vi "Start Acquisition and Logging.vi"(8 "error in (no error)":errorcluster, 11 "Acquisition and Logging Configuration":T1={"Data Rate"=1, "Samples per Read"=0, "Number of Reads to Save"=0, "Data File Name"="", "TDMS Properties"=[], "Number of Channels"=4, "Channel Scale Array"=[0.0, 0.0, 0.0, 0.0], "Channel Names"=[], "Trigger - RMS Value"=0.0, "Trigger - Channel"=0, "Trigger - Time (Minute)"=0} {"Data Rate" items=["51.200 kS/s (NI 9234)"=1, "25.600 kS/s (NI 9234)"=2, "17.067 kS/s (NI 9234)"=3, "12.800 kS/s (NI 9234)"=4, "10.240 kS/s (NI 9234)"=5, "8.533 kS/s (NI 9234)"=6, "7.314 kS/s (NI 9234)"=7, "6.400 kS/s (NI 9234)"=8, "5.689 kS/s (NI 9234)"=9, "5.120 kS/s (NI 9234)"=10, "4.654 kS/s (NI 9234)"=11, "4.267 kS/s (NI 9234)"=12, "3.938 kS/s (NI 9234)"=13, "3.657 kS/s (NI 9234)"=14, "3.413 kS/s (NI 9234)"=15, "3.200 kS/s (NI 9234)"=16, "3.012 kS/s (NI 9234)"=17, "2.845 kS/s (NI 9234)"=18, "2.695 kS/s (NI 9234)"=19, "2.560 kS/s (NI 9234)"=20, "2.438 kS/s (NI 9234)"=21, "2.328 kS/s (NI 9234)"=22, "2.226 kS/s (NI 9234)"=23, "2.133 kS/s (NI 9234)"=24, "2.048 kS/s (NI 9234)"=25, "1.969 kS/s (NI 9234)"=26, "1.896 kS/s (NI 9234)"=27, "1.829 kS/s (NI 9234)"=28, "1.765 kS/s (NI 9234)"=29, "1.707 kS/s (NI 9234)"=30, "1.652 kS/s (NI 9234)"=31]}) -> (0 "error out":errorcluster, 1 "Wait on IRQ Timeout?":bool, 2 "Total Buffer Size":i32, 3 "FPGA VI Reference Out":T4)   [LabVIEW 2020]
uses:
  controls/FPGA VI Reference.ctl
  controls/Acquisition and Logging Configuration.ctl
  <vilib>/LabVIEW Targets/FPGA/cRIO/shared/nicrio_ModuleControls/nicrio_cRIO-9234_DataRatesRing2.ctl
  controls/TDMS Properties.ctl
  <vilib>/FPGAPlugInAG/cRIO-9038/niLvFpga_Open_cRIO-9038.vi
  <vilib>/FPGAPlugInAG/cRIO-9038/niLvFpga_Reset_cRIO-9038.vi
  <vilib>/Utility/error.llb/Error Cluster From Error Code.vi
  <vilib>/rvi/errors/niLvFpgaAdjustHostInterfaceError.vi
  <vilib>/rvi/interface/common/niFpgaWaitOnOcc.vi
  <vilib>/FPGAPlugInAG/cRIO-9038/niLvFpga_Run_cRIO-9038.vi
  <vilib>/RVI Host/nirviSupport.llb/nirviErrorClusterFromErrorCode.vi
  <vilib>/rvi/interface/nirviOpenFPGA/nirviOpenFPGA.xnode
  FPGA Bitfiles/forthexerciseemc_FPGATarget2_FPGAMain_eC4Nf+bThbM.lvbitx
  FPGA Main.vi
  <vilib>/rvi/interface/nirviMethod/nirviMethod.xnode
  <vilib>/rvi/interface/nirviReadWriteControl/nirviReadWriteControl.xnode
  <vilib>/rvi/errors/niLvFpgaMergeErrorWithErrorCode.vi
  NiFpgaLv.dll
  <vilib>/FPGAPlugInAG/cRIO-9038/niLvFpga_ConfigureFifo_cRIO-9038.vi
  <vilib>/FPGAPlugInAG/cRIO-9038/niLvFpga_StartFifo_cRIO-9038.vi
  <vilib>/rvi/interface/nirviMethod/StockFPGA_InlinedMethodWaitForSingleIRQ.vi
  <vilib>/FPGAPlugInAG/cRIO-9038/niLvFpga_WaitOnIrq_cRIO-9038.vi
  <vilib>/FPGAPlugInAG/cRIO-9038/niLvFpga_AcknowledgeIrq_cRIO-9038.vi
panel:
  out "Actual Depth":u32
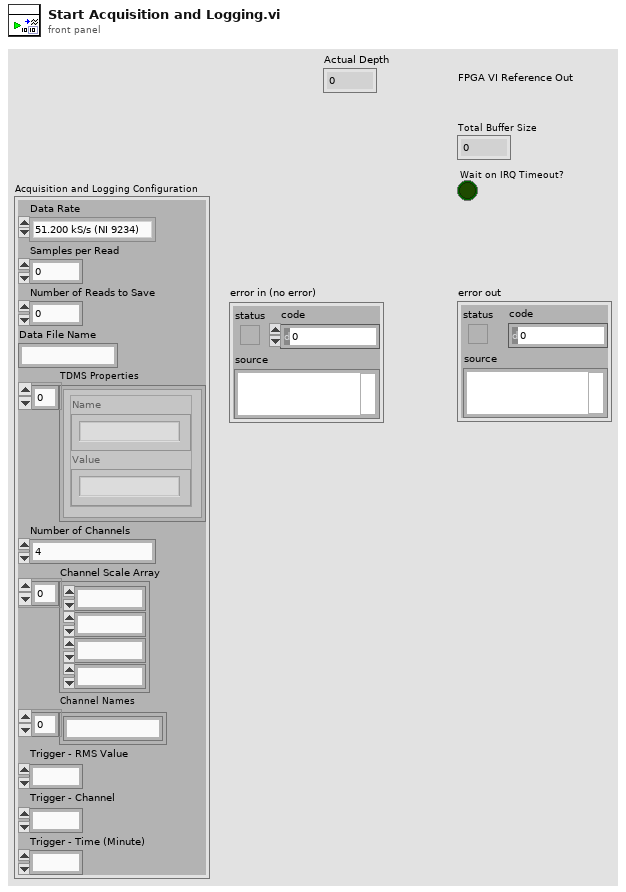
[diagram p1: front panel]
types:
  T1 = typedef "Acquisition and Logging Configuration.ctl" = cluster{"Data Rate":T2, "Samples per Read":i32, "Number of Reads to Save":i32, "Data File Name":string, "TDMS Properties":T3[], "Number of Channels":i32, "Channel Scale Array":fxp<+,24,12>[], "Channel Names":string[], "Trigger - RMS Value":dbl, "Trigger - Channel":i32, "Trigger - Time (Minute)":i32}
  T2 = typedef "nicrio_cRIO-9234_DataRatesRing2.ctl" = u8
  T3 = typedef "TDMS Properties.ctl" = cluster{"Name":string, "Value":string}
  T4 = typedef "FPGA VI Reference.ctl" = refnum<k20>
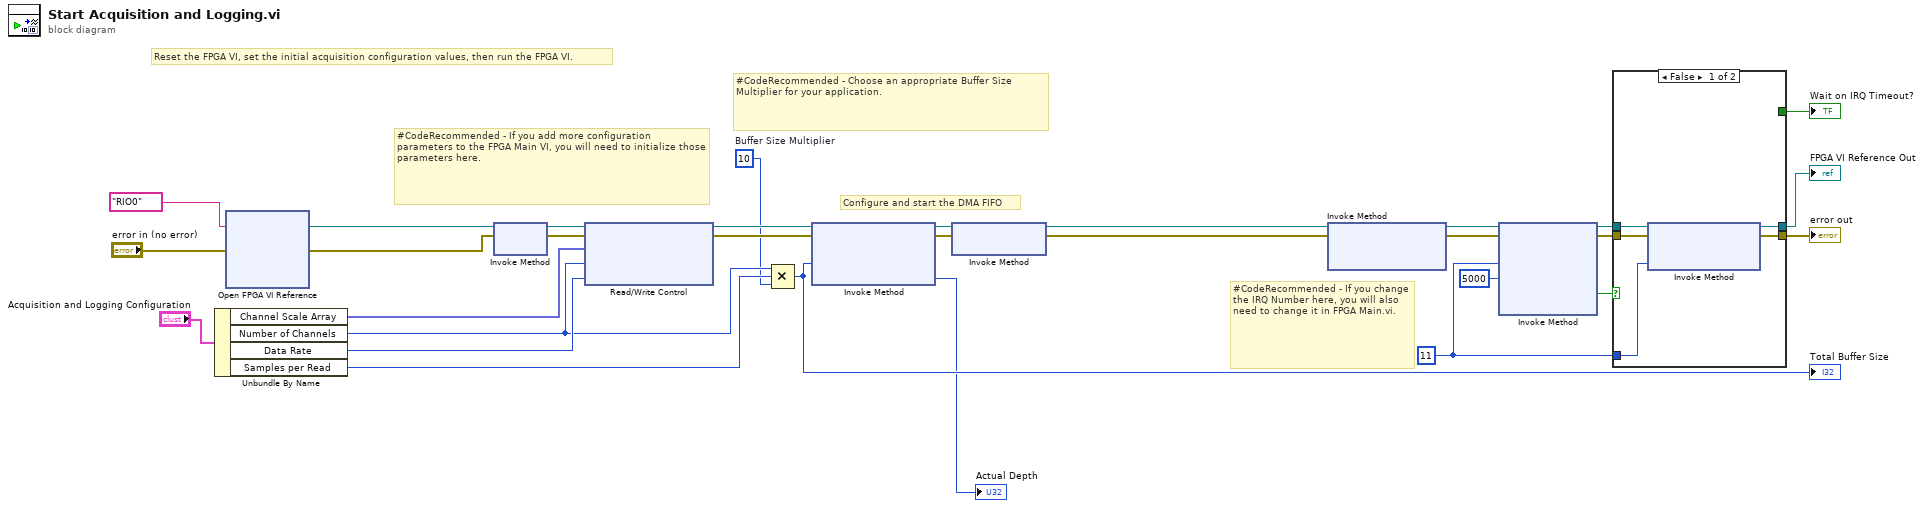
[diagram p0: block diagram]
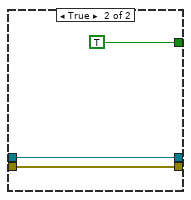
[diagram p2: hidden frame]
diagram:
  w9 = 11
  w10 = 10  # Buffer Size Multiplier
  # "#CodeRecommended - If you change the IRQ Number here, you will also need to change it in FPGA Main.vi."
  # "#CodeRecommended - Choose an appropriate Buffer Size Multiplier for your application."
  # "Configure and start the DMA FIFO"
  # "#CodeRecommended - If you add more configuration parameters to the FPGA Main VI, you will need to initialize those parameters here."
  # "Reset the FPGA VI, set the initial acquisition configuration values, then run the FPGA VI."
  n1 = Unbundle By Name("Acquisition and Logging Configuration") -> ("Channel Scale Array"=w5:fxp<+,24,12>[], "Number of Channels"=w13:i32, "Data Rate"=w19:T2, "Samples per Read"=w12:i32)
  n2 = xnode "Open FPGA VI Reference"("error in"="error in (no error)", "resource name"=tag "RIO0") -> ("FPGA VI Reference Out"=w8:T4, "error out"=w7:errorcluster)
  n3 = xnode "Invoke Method"("FPGA VI Reference In"=w8, "error in"=w7) -> ("FPGA VI Reference Out"=w27:T4, "error out"=w26:errorcluster)
  n4 = xnode "Read/Write Control"("FPGA VI Reference In"=w27, "error in"=w26, "Channel Scale Array"=w5, "Number of Channels"=w13, "Data Rate"=w19) -> ("FPGA VI Reference Out"=w15:T4, "error out"=w14:errorcluster)
  n5 = Compound Arithmetic op=MULTIPLY(w13, w12, w10) -> (w11:i32)
  "Total Buffer Size" <- w11
  n6 = xnode "Invoke Method"("FPGA VI Reference In"=w15, "error in"=w14, "Requested Depth"=w11) -> ("FPGA VI Reference Out"=w16:T4, "error out"=w17:errorcluster, "Actual Depth"=→"Actual Depth":u32)
  n7 = xnode "Invoke Method"("FPGA VI Reference In"=w16, "error in"=w17) -> ("FPGA VI Reference Out"=w1:T4, "error out"=w2:errorcluster)
  n8 = xnode "Invoke Method"("FPGA VI Reference In"=w1, "error in"=w2) -> ("FPGA VI Reference Out"=w28:T4, "error out"=w29:errorcluster)  [unwired: 1 in]
  n9 = xnode "Invoke Method"("FPGA VI Reference In"=w28, "error in"=w29, "IRQ Number(s)"=w9, "Timeout (ms)"=5000) -> ("FPGA VI Reference Out"=w20:T4, "error out"=w21:errorcluster, "Timed Out"=w23:bool)  [unwired: 1 out]
  n10 = case shown="False" w23 {
    tunnel: w20 -> [w35 w36]
    tunnel: w21 -> [w34 w38]
    tunnel: [w33 w38] -> w24
    tunnel: w9 -> [w32 _]
    tunnel: [_ TRUE] -> w25
    tunnel: [w31 w36] -> w30
    frame False {
      n11 = xnode "Invoke Method"("FPGA VI Reference In"=w35, "error in"=w34, "IRQ Number(s)"=w32) -> ("FPGA VI Reference Out"=w31:T4, "error out"=w33:errorcluster)
    }
    frame True {
    }
  }
  "FPGA VI Reference Out" <- w30
  "Wait on IRQ Timeout?" <- w25
  "error out" <- w24
